vi "WL_Joystick RT Driver VI.vi"(7 "Operation":T1, 11 "Device Reference in":T2 format="%.0x") -> (0 "Error Code":i32)   [LabVIEW 2014, in "WL_Joystick Custom Device.lvlib"]
uses:
  WL_Joystick Custom Device.lvlib
  <vilib>/NI Veristand/Custom Device API/Custom Device Item Ref.ctl
  <vilib>/NI Veristand/Custom Device API/Hardware Interface Driver VI Operation.ctl
  <vilib>/NI Veristand/Custom Device API/Custom Device Channel Type.ctl
  <vilib>/NI Veristand/Custom Device API/Data Reference.ctl
  <vilib>/NI Veristand/Custom Device API/Block Data Reference.ctl
  <vilib>/NI Veristand/Custom Device API/Data Access Type.ctl
  <vilib>/NI Veristand/Custom Device Tools/Custom Device Utility Library/RT Debug String Color Spec.ctl
  GlobalGUI.vi
  <vilib>/NI Veristand/Custom Device API/Get Item Property (String).vi
  <vilib>/NI Veristand/Custom Device API/Get Item Property (U16).vi
  <vilib>/NI Veristand/Custom Device API/Global Data Refs.vi
  <vilib>/NI Veristand/Custom Device API/Custom Device API.lvlib
  <vilib>/NI Veristand/Custom Device Tools/Custom Device Utility Library/Custom Device Utility Library.lvlib
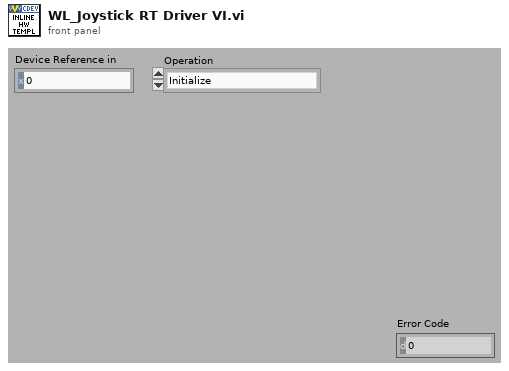
[diagram p1: front panel]
types:
  T1 = typedef "Custom Device API.lvlib/Hardware Interface Driver VI Operation.ctl" = enum16{"Initialize", "Start", "Read Data from HW", "Write Data to HW", "Close"}
  T2 = typedef "Custom Device API.lvlib/Custom Device Item Ref.ctl" = u64
  T3 = typedef "Custom Device API.lvlib/Data Reference.ctl" = i32
  T4 = typedef "Custom Device API.lvlib/Block Data Reference.ctl" = cluster{"Data Reference":T3, "Offset":i32, "Length":i32}
  T5 = cluster{"Input Values":dbl[], "Input Refs":T3[], "Output Values":dbl[], "Output Refs":T3[], "Device Error":errorcluster, "connection ID":refnum<k5>, "InputRefs":T4[], "OutputRefs":T4[]}
  T6 = typedef "Custom Device API.lvlib/Data Access Type.ctl" = enum16{"Read", "Write"}
  T7 = typedef "Custom Device API.lvlib/Custom Device Channel Type.ctl" = enum16{"Input", "Output"}
  T8 = enum16{"Standard", "Buffered", "CRLF", "Immediate"}
  T9 = typedef "Custom Device Utility Library.lvlib/RT Debug String Color Spec.ctl" = u16
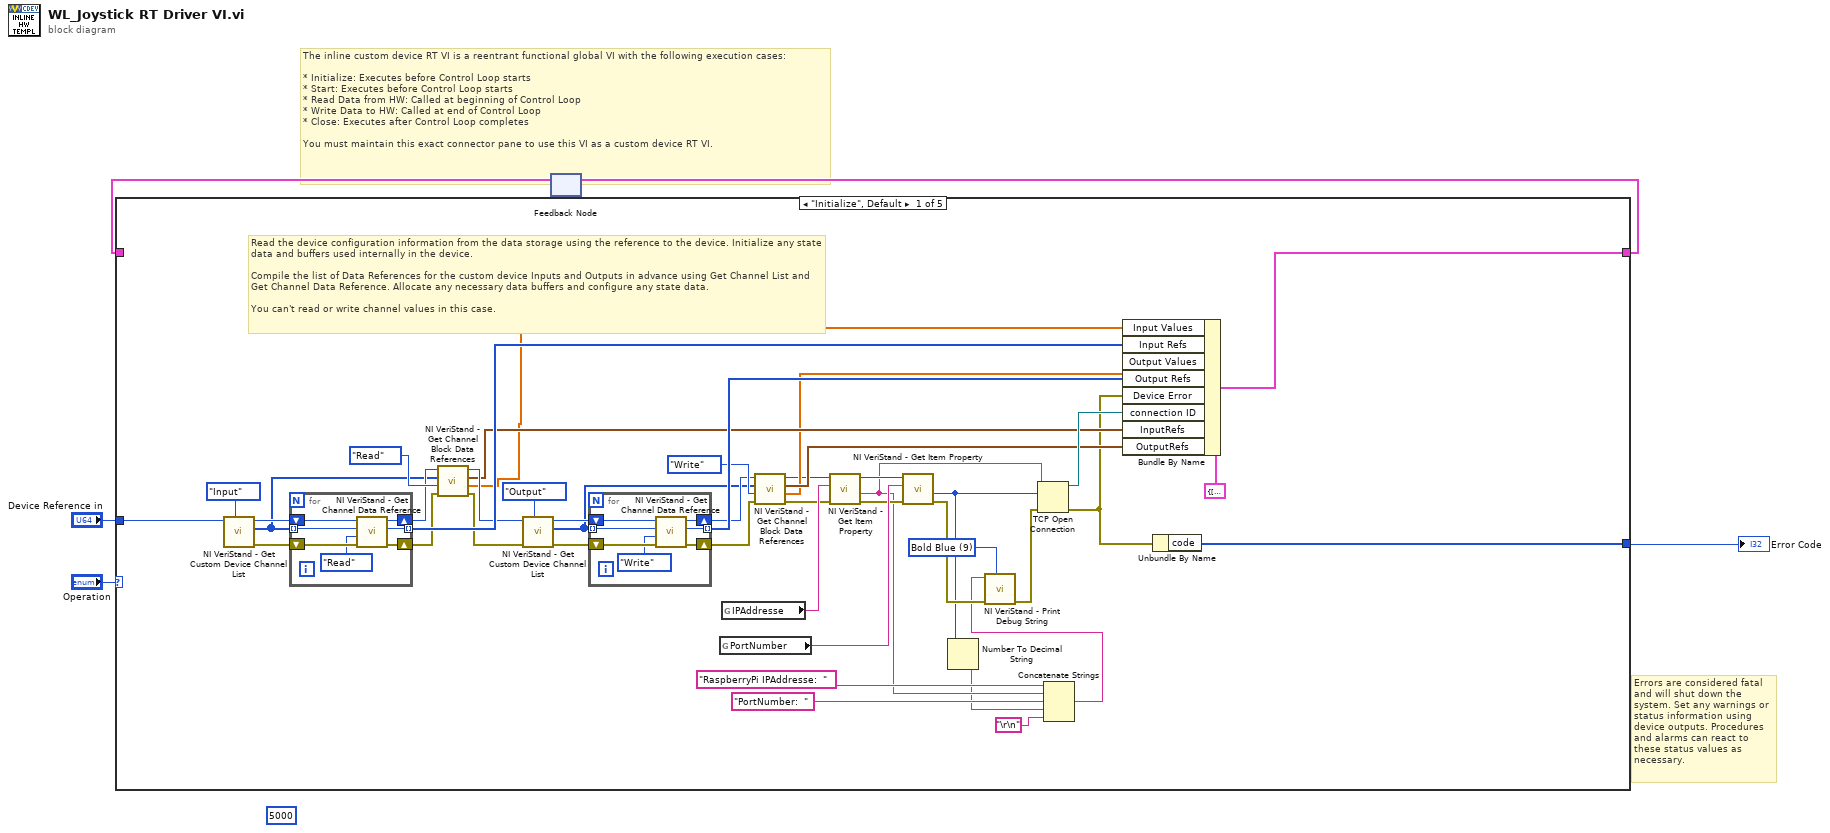
[diagram p0: block diagram]
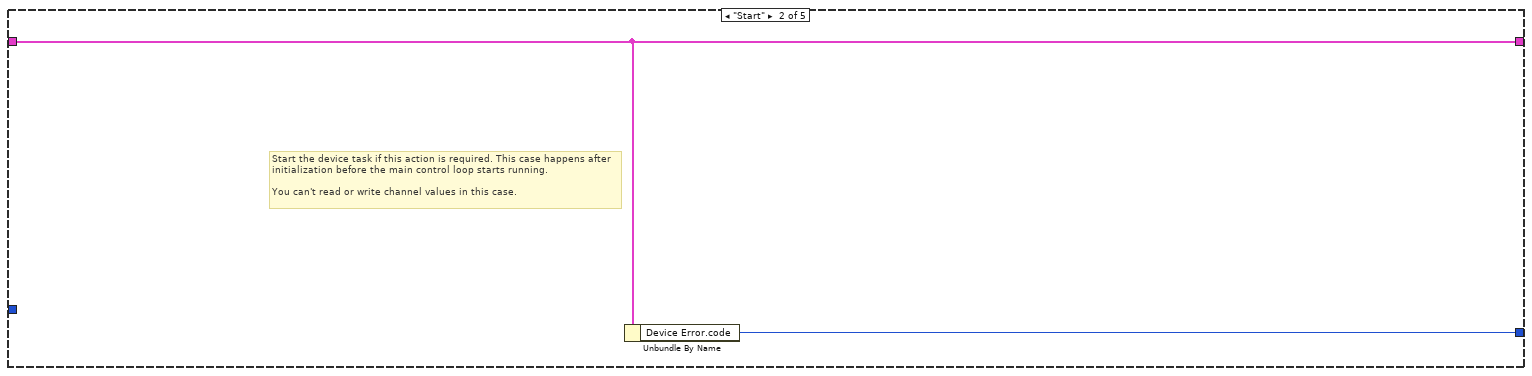
[diagram p2: hidden frame]
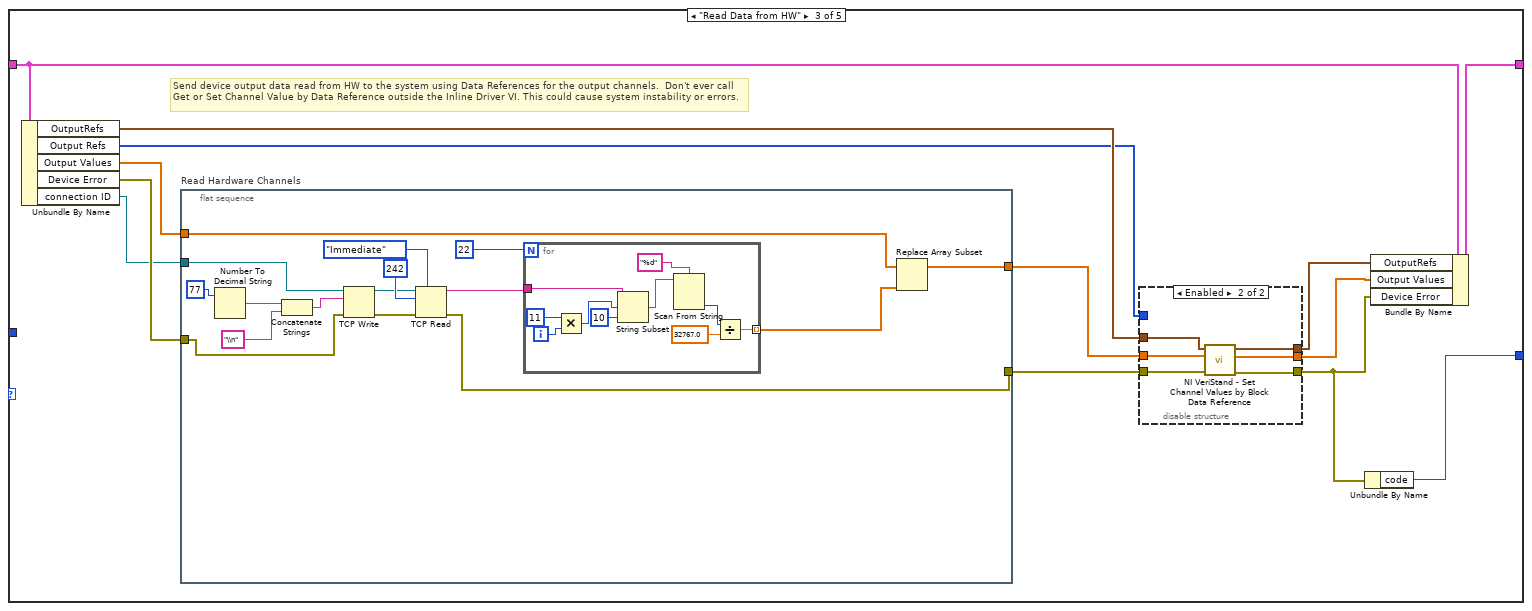
[diagram p3: hidden frame]
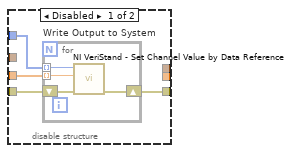
[diagram p4: hidden frame]
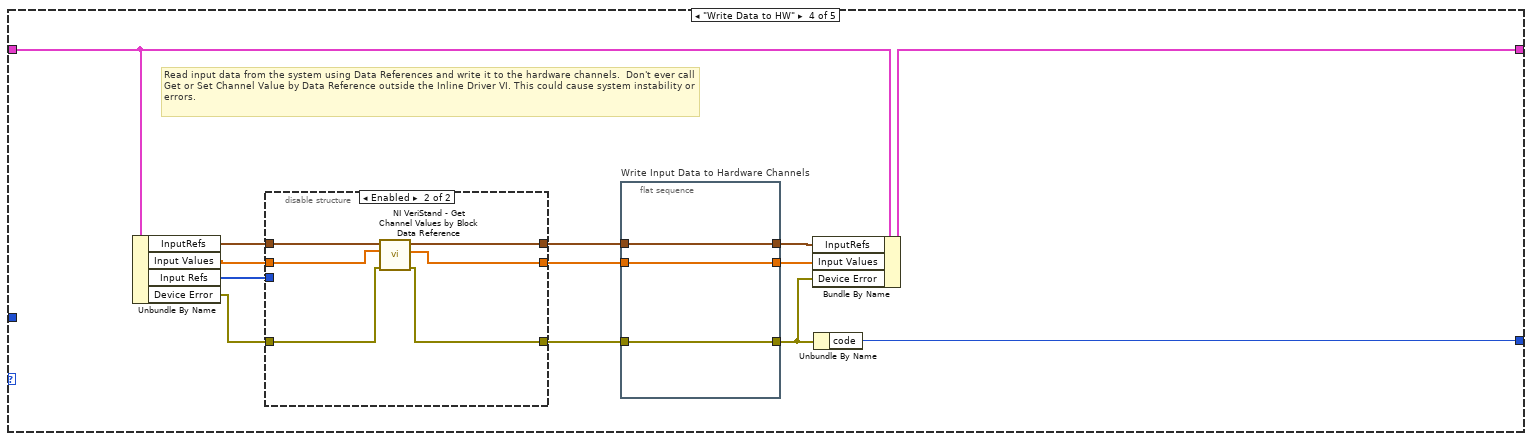
[diagram p5: hidden frame]
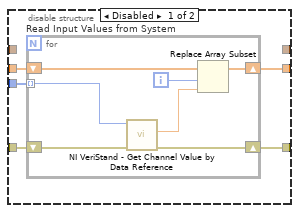
[diagram p6: hidden frame]
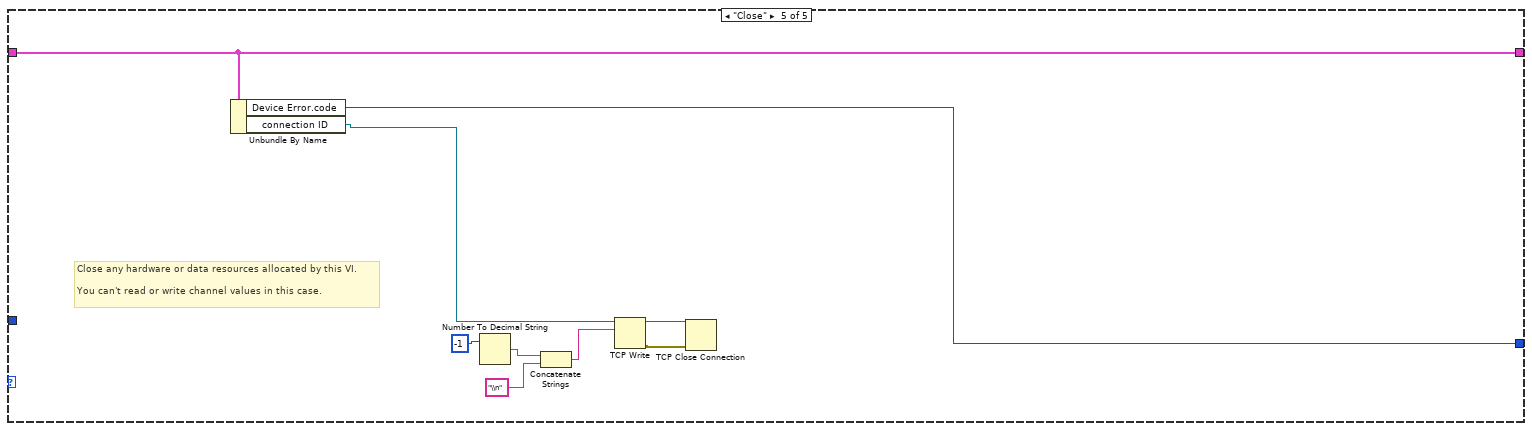
[diagram p7: hidden frame]
diagram:
  (unwired) 5000 ("timeout ms (25000)")
  # "Errors are considered fatal and will shut down the system. Set any warnings or status information using device outputs. Procedures and alarms can react to these status values as necessary."
  # "The inline custom device RT VI is a reentrant functional global VI with the following execution cases:\n\n* Initialize: Executes before Control Loop starts\n* Start: Executes before Control Loop starts\n* Read Data from HW: Called at beginning of Control Loop\n* Write Data to HW: Called at end of Control Loop\n* Close: Executes after Control Loop completes\n\nYou must maintain this exact connector pane to use this VI as a custom device RT VI."
  n1 = feedback #1() -> (w3:T5)  [unwired: 1 out]
  n2 = case shown="\"Initialize\", Default" "Operation" {
    tunnel: [w47 w64 w76 w130 w160] -> w4
    tunnel: w3 -> [_ w64 w77 w131 w160]
    tunnel: "Device Reference in" -> [w48 _ _ _ _]
    tunnel: [w46 w65 w66 w128 w161] -> w1
    frame "Initialize", Default {
      w6 = T9 9 items=["Plain White"=7, "Bold White"=15, "Bold Blue"=9, "Bold Green"=10, "Bold Red"=12] ("Attribute")
      # "Read the device configuration information from the data storage using the reference to the device. Initialize any state data and buffers used internally in the device.\n\nCompile the list of Data References for the custom device Inputs and Outputs in advance using Get Channel List and Get Channel Data Reference. Allocate any necessary data buffers and configure any state data.\n\nYou can't read or write channel values in this case."
      n3 = call <vilib>:"NI VeriStand - Get Custom Device Channel List.vi"("Channel Type"=Custom_Device_Channel_Type."Input", "Device Ref in"=w48) -> ("error out"=w44:errorcluster, "Specified Channel Ref List"=w29:T2[], "Device Ref out"=w45:T2)  [unwired: 1 in, 6 out]
      n4 = for {
        shift-right: [w58] -> w34
        shift-left: w45 -> [w62]
        tunnel: w29 -> [w61] mode=indexing
        shift-right: [w59] -> w31
        shift-left: w44 -> [w63]
        tunnel: [w57] -> w40 mode=indexing
        n5 = call <vilib>:"NI VeriStand - Get Channel Data Reference.vi"("error in (no error)"=w63, "Access"=Data_Access_Type."Read", "Channel Ref in"=w61, "Device Ref in"=w62) -> ("error out"=w59:errorcluster, "Channel Data Reference"=w57:T3, "Device Ref out"=w58:T2)  [unwired: 5 out]
      }
      n6 = call <vilib>:"NI VeriStand - Get Channel Block Data References.vi"("error in (no error)"=w31, "Access"=Data_Access_Type."Read", "Channel Refs"=w29, "Device Ref in"=w34) -> ("error out"=w30:errorcluster, "Values Array"=w26:dbl[], "Block Data Refs"=w28:T4[], "Device Ref out"=w33:T2)  [unwired: 4 in]
      n7 = call <vilib>:"NI VeriStand - Get Custom Device Channel List.vi"("Channel Type"=Custom_Device_Channel_Type."Output", "error in (no error)"=w30, "Device Ref in"=w33) -> ("error out"=w43:errorcluster, "Specified Channel Ref List"=w24:T2[], "Device Ref out"=w42:T2)  [unwired: 6 out]
      n8 = for {
        tunnel: w24 -> [w54] mode=indexing
        shift-right: [w52] -> w23
        shift-left: w43 -> [w56]
        tunnel: [w51] -> w39 mode=indexing
        shift-right: [w50] -> w32
        shift-left: w42 -> [w55]
        n9 = call <vilib>:"NI VeriStand - Get Channel Data Reference.vi"("error in (no error)"=w56, "Access"=Data_Access_Type."Write", "Channel Ref in"=w54, "Device Ref in"=w55) -> ("error out"=w52:errorcluster, "Channel Data Reference"=w51:T3, "Device Ref out"=w50:T2)  [unwired: 5 out]
      }
      n10 = global read "GlobalGUI.vi" "PortNumber"() -> (w18:string)
      n11 = global read "GlobalGUI.vi" "IPAddresse"() -> (w22:string)
      n12 = call <vilib>:"NI VeriStand - Get Channel Block Data References.vi"("error in (no error)"=w23, "Access"=Data_Access_Type."Write", "Channel Refs"=w24, "Device Ref in"=w32) -> ("error out"=w20:errorcluster, "Values Array"=w25:dbl[], "Block Data Refs"=w27:T4[], "Device Ref out"=w21:T2)  [unwired: 4 in]
      n13 = call-poly <vilib>:"NI VeriStand - Get Item Property.vi"("error in (no error)"=w20, "Property Name"=w22, "Item Ref in"=w21) -> ("error out"=w17:errorcluster, "Value"=w12:string, "Item Ref out"=w19:T2)  [unwired: 5 in, 1 out]
      n14 = call-poly <vilib>:"NI VeriStand - Get Item Property.vi"("error in (no error)"=w17, "Property Name"=w18, "Item Ref in"=w19) -> ("error out"=w15:errorcluster, "Value"=w10:u16)  [unwired: 5 in, 2 out]
      n15 = Number To Decimal String(number=w10) -> (decimal integer string=w9:string)  [unwired: 1 in]
      n16 = Concatenate Strings("RaspberryPi IPAddresse:  " ("string"), w12, "PortNumber:  " ("string"), w9, "\r\n") -> (w7:string)
      n17 = call <vilib>:"NI VeriStand - Print Debug String.vi"("Attribute"=w6, "error in (no error)"=w15, "Message"=w7) -> ("error out"=w14:errorcluster)  [unwired: 8 in]
      n18 = TCP Open Connection(address=w12, remote port or service name=w10, error in (no error)=w14) -> (connection ID=w37:refnum<k5>, error out=w16:errorcluster)  [unwired: 2 in]
      n19 = Bundle By Name(cluster=T5 {"Input Values"=[], "Input Refs"=[], "Output Values"=[], "Output Refs"=[], "Device Error"={"status"=FALSE, "code"=0, "source"=""}, "connection ID"=refnum, "InputRefs"=[], "OutputRefs"=[]}, "Input Values"=w26, "Input Refs"=w40, "Output Values"=w25, "Output Refs"=w39, "Device Error"=w16, "connection ID"=w37, "InputRefs"=w28, "OutputRefs"=w27) -> (w47:T5)
      n20 = Unbundle By Name(w16) -> ("code"=w46:i32)
    }
    frame "Start" {
      # "Start the device task if this action is required. This case happens after initialization before the main control loop starts running.\n\nYou can't read or write channel values in this case."
      n21 = Unbundle By Name(w64) -> ("Device Error.code"=w65:i32)
    }
    frame "Read Data from HW" {
      # "Send device output data read from HW to the system using Data References for the output channels.  Don't ever call Get or Set Channel Value by Data Reference outside the Inline Driver VI. This could cause system instability or errors."
      n22 = Unbundle By Name(w77) -> ("OutputRefs"=w70:T4[], "Output Refs"=w69:T3[], "Output Values"=w78:dbl[], "Device Error"=w75:errorcluster, "connection ID"=w74:refnum<k5>)
      n23 = flat-sequence "Read Hardware Channels" {
        tunnel: w75 -> [w83]
        tunnel: [w81] -> w71
        tunnel: [w93] -> w72
        tunnel: w78 -> [w94]
        tunnel: w74 -> [w84]
        frame #0 {
          n24 = Number To Decimal String(number=77) -> (decimal integer string=w88:string)  [unwired: 1 in]
          n25 = Concatenate Strings(w88, "\\n" ("string")) -> (w86:string)
          n26 = TCP Write(connection ID=w84, data in=w86, error in (no error)=w83) -> (connection ID out=w91:refnum<k5>, error out=w90:errorcluster)  [unwired: 1 in, 1 out]
          n27 = TCP Read(connection ID=w91, bytes to read=242, error in (no error)=w90, 7:T8."Immediate" ("mode (standard)")) -> (data out=w79:string, error out=w81:errorcluster)  [unwired: 1 in, 1 out]
          n28 = for {
            N: 22 -> [_]
            tunnel: w79 -> [w104]
            tunnel: [w96] -> w82 mode=indexing
            i -> [w102]
            n29 = Multiply(x=11, y=w102) -> (x*y=w100:i32)
            n30 = String Subset(string=w104, offset (0)=w100, length (rest)=10 ("length (rest)")) -> (substring=w99:string)
            n31 = Scan From String(format string="%d", input string=w99) -> (output 1=w95:i32)  [unwired: 3 in, 3 out]
            n32 = Divide(x=w95, y=32767.0) -> (x/y=w96:dbl)
          }
          n33 = Replace Array Subset(array=w94, new element=w82) -> (w93:dbl[])  [unwired: 1 in]
        }
      }
      n34 = disable-structure shown="Enabled" {
        disable-tunnel: w71 -> [w108 w114]
        disable-tunnel: w69 -> [w107 _]
        disable-tunnel: [w106 w118] -> w67
        disable-tunnel: w72 -> [w105 w113]
        disable-tunnel: [_ w117] -> w68
        disable-tunnel: [_ w116] -> w73
        disable-tunnel: w70 -> [_ w115]
        frame Disabled {
          n35 = for "Write Output to System" {
            shift-right: [w111] -> w106
            shift-left: w108 -> [w112]
            tunnel: w105 -> [w110] mode=indexing
            tunnel: w107 -> [w109] mode=indexing
            n36 = call <vilib>:"NI VeriStand - Set Channel Value by Data Reference.vi"("error in (no error)"=w112, "Value"=w110, "Data Reference in"=w109) -> ("error out"=w111:errorcluster)  [unwired: 8 out]
          }
        }
        frame Enabled {
          n37 = call <vilib>:"NI VeriStand - Set Channel Values by Block Data Reference.vi"("error in (no error)"=w114, "Values Array in"=w113, "Block Data Ref"=w115) -> ("error out"=w118:errorcluster, "Values Array out"=w117:dbl[], "Block Data Ref dup"=w116:T4[])  [unwired: 6 in]
        }
      }
      n38 = Unbundle By Name(w67) -> ("code"=w66:i32)
      n39 = Bundle By Name(cluster=w77, "OutputRefs"=w73, "Output Values"=w68, "Device Error"=w67) -> (w76:T5)
    }
    frame "Write Data to HW" {
      # "Read input data from the system using Data References and write it to the hardware channels.  Don't ever call Get or Set Channel Value by Data Reference outside the Inline Driver VI. This could cause system instability or errors."
      n40 = Unbundle By Name(w131) -> ("InputRefs"=w126:T4[], "Input Values"=w125:dbl[], "Input Refs"=w124:T3[], "Device Error"=w123:errorcluster)
      n41 = disable-structure shown="Enabled" {
        disable-tunnel: w124 -> [w136 _]
        disable-tunnel: w125 -> [w135 w147]
        disable-tunnel: [w134 w146] -> w122
        disable-tunnel: [w133 w144] -> w121
        disable-tunnel: w123 -> [w132 w145]
        disable-tunnel: w126 -> [_ w149]
        disable-tunnel: [_ w148] -> w119
        frame Disabled {
          n42 = for "Read Input Values from System" {
            shift-right: [w137] -> w133
            shift-left: w132 -> [w143]
            tunnel: w136 -> [w142] mode=indexing
            shift-right: [w140] -> w134
            shift-left: w135 -> [w141]
            i -> [w139]
            n43 = call <vilib>:"NI VeriStand - Get Channel Value by Data Reference.vi"("error in (no error)"=w143, "Data Reference in"=w142) -> ("error out"=w137:errorcluster, "Value"=w138:dbl)  [unwired: 8 out]
            n44 = Replace Array Subset(array=w141, new element=w138, index=w139) -> (w140:dbl[])
          }
        }
        frame Enabled {
          n45 = call <vilib>:"NI VeriStand - Get Channel Values by Block Data Reference.vi"("error in (no error)"=w145, "Values Array in"=w147, "Block Data Ref"=w149) -> ("error out"=w144:errorcluster, "Values Array out"=w146:dbl[], "Block Data Ref dup"=w148:T4[])  [unwired: 6 in]
        }
      }
      n46 = flat-sequence "Write Input Data to Hardware Channels" {
        tunnel: w122 -> [w152]
        tunnel: [w152] -> w129
        tunnel: [w151] -> w127
        tunnel: w121 -> [w151]
        tunnel: [w150] -> w120
        tunnel: w119 -> [w150]
        frame #0 {
        }
      }
      n47 = Bundle By Name(cluster=w131, "InputRefs"=w120, "Input Values"=w129, "Device Error"=w127) -> (w130:T5)
      n48 = Unbundle By Name(w127) -> ("code"=w128:i32)
    }
    frame "Close" {
      # "Close any hardware or data resources allocated by this VI.\n\nYou can't read or write channel values in this case."
      n49 = Unbundle By Name(w160) -> ("Device Error.code"=w161:i32, "connection ID"=w159:refnum<k5>)
      n50 = Number To Decimal String(number=-1) -> (decimal integer string=w157:string)  [unwired: 1 in]
      n51 = Concatenate Strings(w157, "\\n" ("string")) -> (w155:string)
      n52 = TCP Write(connection ID=w159, data in=w155) -> (connection ID out=w153:refnum<k5>, error out=w154:errorcluster)  [unwired: 2 in, 1 out]
      n53 = TCP Close Connection(connection ID=w153, error in (no error)=w154) -> ()  [unwired: 1 in, 2 out]
    }
  }
  "Error Code" <- w1
  n54 = feedback-in #1(w4) -> ()
